vi "LRC-接收校验.vi"(11 "完整输入":string) -> (0 "LRC？":bool, 3 "净数据":string)   [LabVIEW 2013]
panel:
  out "LRC":string
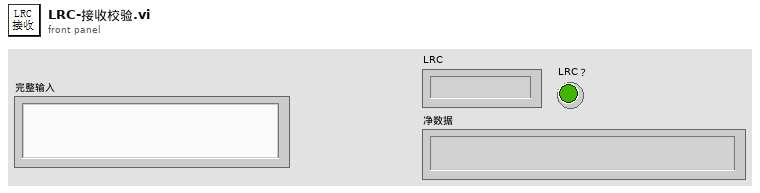
[diagram p1: front panel]
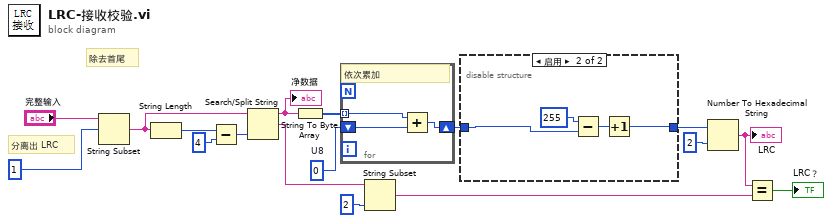
[diagram p0: block diagram]
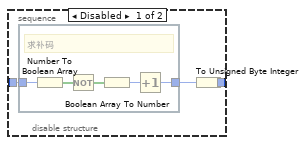
[diagram p2: hidden frame]
diagram:
  w17 = u8 0  # U8
  # "分离出 LRC"
  # "除去首尾"
  n1 = String Subset(string="完整输入", offset (0)=1 ("偏移量(0)")) -> (substring=w13:string)  [unwired: 1 in]
  n2 = String Length(string=w13) -> (length=w11:i32)
  n3 = Subtract(x=w11, y=4 ("偏移量(0)")) -> (x-y=w10:i32)
  n4 = Search/Split String(string=w13, offset (0)=w10) -> (substring before match=w9:string, match + rest of string=w8:string)  [unwired: 1 in, 1 out]
  "净数据" <- w9
  n5 = String To Byte Array(string=w9) -> (unsigned byte array=w5:u8[])
  n6 = for {
    shift-right: [w20] -> w4
    shift-left: w17 -> [w19]
    tunnel: w5 -> [w18] mode=indexing
    # "依次累加"
    n7 = Add(x=w18, y=w19) -> (x+y=w20:u8)
  }
  n8 = String Subset(string=w8, length (rest)=2 ("长度（剩余）")) -> (substring=w6:string)  [unwired: 1 in]
  n9 = disable-structure shown="启用" {
    disable-tunnel: w4 -> [w23 w30]
    disable-tunnel: [w21 w29] -> w3
    frame Disabled {
      n10 = stacked-sequence {
        tunnel: w23 -> [w28]
        tunnel: [w24] -> w22
        frame #0 {
          # "求补码"
          n11 = Number To Boolean Array(number=w28) -> (Boolean array=w27:bool[])
          n12 = Not(x=w27) -> (.not. x?=w26:bool[])
          n13 = Boolean Array To Number(Boolean array=w26) -> (number=w25:u32)
          n14 = Increment(x=w25) -> (x+1=w24:u32)
        }
      }
      n15 = To Unsigned Byte Integer(number=w22) -> (unsigned 8bit integer=w21:u8)
    }
    frame Enabled {
      n16 = Subtract(x=u8 255 ("无符号16位整型"), y=w30) -> (x-y=w31:u8)
      n17 = Increment(x=w31) -> (x+1=w29:u8)
    }
  }
  n18 = Number To Hexadecimal String(1:i16 2 ("宽度(-)"), 2:w3) -> (0:w1:string)
  "LRC" <- w1
  n19 = Equal?(x=w1, y=w6) -> (x = y?=→"LRC？":bool)
